vi "Obtain ref source ctrl value.vi"() -> (2 "select_ref_red":bool)   [LabVIEW 2020]
uses:
  Global Variables/gl_UI Ctrl Refs.vi
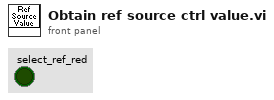
[diagram p1: front panel]
types:
  T1 = typedef "UI ctrl refs cluster.ctl" = cluster{"Top level VI path":path, "Top level VI ref":refnum<vi>, "User menu ref":refnum<k9>, "Sub Panel control":refnum<vi>, "Imaging Param Tab":refnum<vi>, "Occurrence-Start drivers":refnum<k4>, "Occurrence-Speed logging initialised":refnum<k4>, "Occurrence-XYZ stage initialised":refnum<k4>, "Exit button":refnum<vi>, "Status ind":refnum<vi>, "Set as origin":refnum<vi>, "Speed Logging":refnum<vi>, "Time Lapse":refnum<vi>, "Live Imaging":refnum<vi>, "AOL Z Stack":refnum<vi>, "Motor Z Stack":refnum<vi>, "Funct Acq button":refnum<vi>, "Hard Shutter":refnum<vi>, "Virtual Shutter":refnum<vi>, "Laser Power":refnum<vi>, "AOL Mode":refnum<vi>, "Frame Size":refnum<vi>, "Field of View":refnum<vi>, "Dwell Time":refnum<vi>, "Zoom":refnum<vi>, "AOL Z":refnum<vi>, "Objective":refnum<vi>, "Axis":refnum<vi>, "Paths & Names":refnum<vi>, "Experiment folder path (ind.)":refnum<vi>, "Last State (Ind.)":refnum<vi>, "Averages":refnum<vi>, "Angle (degrees)":refnum<vi>, "X centre":refnum<vi>, "Y centre":refnum<vi>, "Plane Mode":refnum<vi>, "# Planes":refnum<vi>, "Z Start":refnum<vi>, "Z Stop":refnum<vi>, "Z Step":refnum<vi>, "PMT 1":refnum<vi>, "PMT 2":refnum<vi>, "Stage XYZ Position":refnum<vi>, "Pockels@Z Start":refnum<vi>, "Pockels@Z Stop":refnum<vi>, "Obtain Z Start":refnum<vi>, "Obtain Z Stop":refnum<vi>, "Live stim.trig.period":refnum<vi>, "Live stim.trig.enable":refnum<vi>, "Movement Correction":refnum<vi>, "Load Reference Image":refnum<vi>, "XY Stage Move":refnum<vi>, "MovCor Cluster":refnum<vi>, "RefDAQParam":refnum<vi>, "Funct. Acq. Pockels Modulation":refnum<vi>, "Ref Laser Power":refnum<vi>, "Enable Video Recording":refnum<vi>, "Video Record-Live Imaging":refnum<vi>, "Video Record-Funct acq":refnum<vi>, "Reference Source":refnum<vi>, "AOL Z-stack Chirps Ready (ind)":refnum<vi>, "Target time between mov.cor. ref triggers (ms)":refnum<vi>, "Funct. Acq. Ref frame save":refnum<vi>, "Tracking button":refnum<vi>, "Show ref plots window":refnum<vi>, "Center freq ind (nm)":refnum<vi>, "Pickup mode (ind)":refnum<vi>, "Logging queue (ind)":refnum<vi>, "Back aperture power (ind.)":refnum<vi>, "Power after objective (ind.)":refnum<vi>, "Switch user":refnum<vi>, "Ls1 Conn. Status":refnum<vi>, "Ls1Tuning Status":refnum<vi>, "Ls1 Faults":refnum<vi>, "Ls1 Connection":refnum<vi>, "Ls1 Mode":refnum<vi>, "Ls1 POWER [mW]":refnum<vi>, "Ls1Shutter":refnum<vi>, "Ls1 Wavelength":refnum<vi>, "Ls1 Note":refnum<vi>, "Ls1 Confirm Wav":refnum<vi>, "Ls1 PreChrp Prism1":refnum<vi>, "Ls1 PreChrp Prism2":refnum<vi>, "Ls1 wav top Ind":refnum<vi>, "Ls1 power top Ind":refnum<vi>, "Ls1 Pump peak Hold":refnum<vi>, "Ls1 Status Ind":refnum<vi>, "Ls1 wav cancel":refnum<vi>, "Experiment Type":refnum<vi>, "Biology Information":refnum<vi>, "Camera recording status":refnum<vi>}
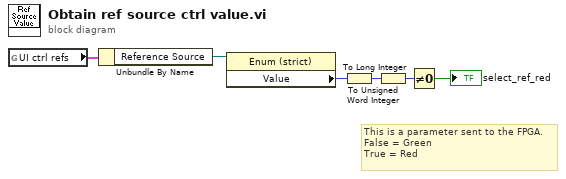
[diagram p0: block diagram]
diagram:
  # "This is a parameter sent to the FPGA.\nFalse = Green\nTrue = Red"
  n1 = global read "gl_UI Ctrl Refs.vi" "UI ctrl refs"() -> (w1:T1)
  n2 = Unbundle By Name(w1) -> ("Reference Source"=w2:refnum<vi>)
  n3 = property class="Enum (strict)"(reference=w2) -> ("Value"=w3:enum16{"Green channel", "Red channel"})  [unwired: 1 in, 2 out]
  n4 = To Unsigned Word Integer(number=w3) -> (unsigned 16bit integer=w4:u16)
  n5 = To Long Integer(number=w4) -> (32bit integer=w5:i32)
  n6 = Not Equal To 0?(x=w5) -> (x != 0?=→"select_ref_red":bool)
